vi "Agilent E363X Series Output DC Volts.vi"() -> ()   [LabVIEW 2010]
doc: "This example shows how to set the output voltage and current limit levels on the power supply. Constant current mode can be achieved by setting the voltage high enough to make the current through the load reach the current limit.\n\n<B>Note:</B> Channel is only used for the E3631 and is ignored for the other models."
uses:
  <instrlib>/Agilent E363X Series/Agilent E363X Series.lvlib
panel:
  in  "Current Limit (1.0 A)":dbl=1.0 format="%.3g"
  out "Actual Current Level (A)":dbl format="%.3g"
  in  "Voltage Level (5.0 V)":dbl=5.0 format="%.3g"
  in  "Channel (1: Channel 1)":i32(ring)=1 items=["Channel 1"=1, "Channel 2"=2, "Channel 3"=3]
  out "Actual Voltage Level (V)":dbl format="%.3g"
  in  "VISA resource name":refnum<visa-resource-name>
  # "(c) 2008 National Instruments.  ALL RIGHTS RESERVED."
  # "Output Settings"
  # "Measurements"
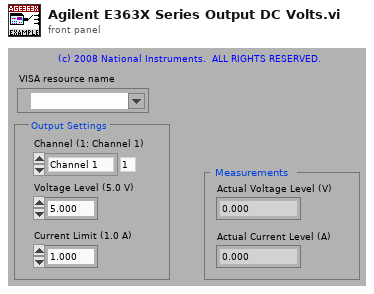
[diagram p1: front panel]
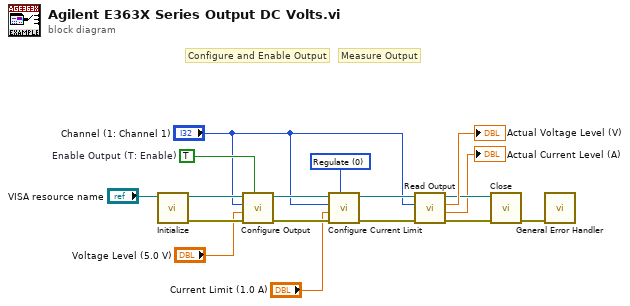
[diagram p0: block diagram]
diagram:
  w1 = u16 0 items=["Regulate", "Trip"] ("Behavior (0: Regulate)")
  w13 = TRUE  # Enable Output (T: Enable)
  # "Measure Output"
  # "Configure and Enable Output"
  n1 = call <instrlib>:"Initialize.vi"("VISA resource name"="VISA resource name") -> ("error out"=w14:errorcluster, "VISA resource name out"=w16:refnum<visa-resource-name>)  [unwired: 9 in]
  n2 = call <instrlib>:"Configure Output.vi"("Enable Output (T: Enable)"=w13, "error in (no error)"=w14, "Voltage Level (0.0 V)"="Voltage Level (5.0 V)", "Channel (1: Channel 1)"="Channel (1: Channel 1)", "VISA resource name"=w16) -> ("error out"=w6:errorcluster, "VISA resource name out"=w7:refnum<visa-resource-name>)  [unwired: 5 in]
  n3 = call <instrlib>:"Configure Current Limit.vi"("Behavior (0: Regulate)"=w1, "error in (no error)"=w6, "Current Limit (0.0 A)"="Current Limit (1.0 A)", "Channel (1: Channel 1)"="Channel (1: Channel 1)", "VISA resource name"=w7) -> ("error out"=w5:errorcluster, "VISA resource name out"=w4:refnum<visa-resource-name>)  [unwired: 5 in]
  n4 = call <instrlib>:"Read Output.vi"("error in (no error)"=w5, "Channel (1: Channel 1)"="Channel (1: Channel 1)", "VISA resource name"=w4) -> ("error out"=w11:errorcluster, "Actual Current Level (A)"=→"Actual Current Level (A)":dbl, "Actual Voltage Level (V)"=→"Actual Voltage Level (V)":dbl, "VISA resource name out"=w10:refnum<visa-resource-name>)  [unwired: 5 in]
  n5 = call <instrlib>:"Close.vi"("error in (no error)"=w11, "VISA resource name"=w10) -> ("error out"=w15:errorcluster)  [unwired: 9 in]
  n6 = call <vilib>:"General Error Handler.vi"("error in (no error)"=w15) -> ()  [unwired: 10 in, 5 out]
